vi "Get RemIO Read Scaling Factor.vi"(8 "error in (no error)":errorcluster, 10 "11120 in":refnum<class "11120.lvclass">, 11 "Node Ptr In":T1 format="%.0x") -> (0 "error out":errorcluster, 1 "Scaling Factors":dbl[](array[numeric]), 2 "11120 out":refnum<class "11120.lvclass">, 3 "Node Ptr Out":T1 format="%.0x", 5 "Per Channel?":bool)   [LabVIEW 2019, in "Modules.lvlib" / "11120.lvclass"]
doc: "This VI Returns the scaling factors for REM IO Input Modules"
uses:
  11120.lvclass
  <vilib>/NI VeriStand/Custom Device API/Custom Device Item Ref.ctl
  11120.lvclass/11120.ctl
  6892548b-0d22-43a4-8def-8bcf3b7e9b02.vi
  RemIO Module/Get RemIO Library Path.vi
  <vilib>/NI VeriStand/Custom Device API/Custom Device API.lvlib
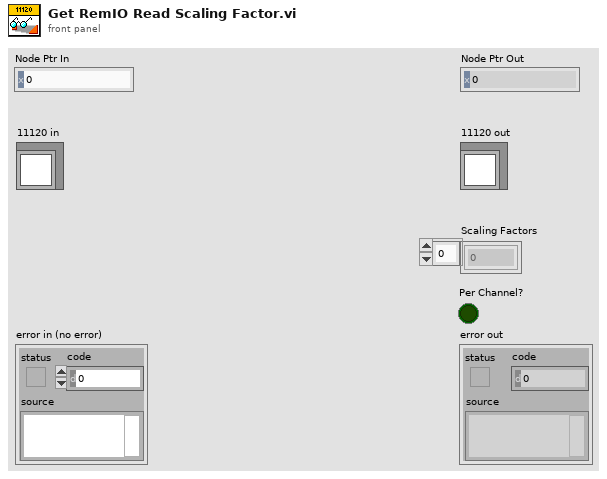
[diagram p1: front panel]
types:
  T1 = typedef "Custom Device API.lvlib/Custom Device Item Ref.ctl" = u64
  T2 = typedef "NI ECAT Remote IO.lvlib/channel number REM-11120.ctl" = u8
  T3 = typedef "NI ECAT Remote IO.lvlib/input filter time REM-11120.ctl" = u8
  T4 = typedef "NI ECAT Remote IO.lvlib/cold junction type REM-11120.ctl" = u8
  T5 = typedef "NI ECAT Remote IO.lvlib/resolution REM-11120.ctl" = u8
  T6 = typedef "NI ECAT Remote IO.lvlib/sensor type REM-11120.ctl" = u8
  T7 = cluster{"channel number":T2, "input filter time":T3, "cold junction type":T4, "resolution":T5, "sensor type":T6}[]
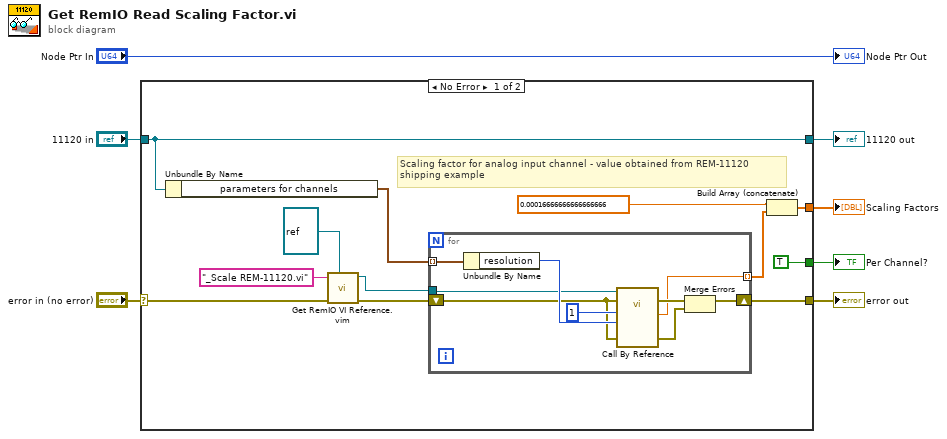
[diagram p0: block diagram]
diagram:
  n1 = case shown="No Error" "error in (no error)" {
    selector: "error in (no error)" -> [w11 w30]
    tunnel: [w18 w30] -> w6
    tunnel: [w17 w29] -> w4
    tunnel: "11120 in" -> [w17 w29]
    tunnel: [w13 _] -> w3
    tunnel: [TRUE _] -> w2
    frame No Error {
      # "Scaling factor for analog input channel - value obtained from REM-11120\nshipping example"
      n2 = Unbundle By Name(w17) -> ("parameters for channels"=w16:T7)
      n3 = call "Get RemIO VI Reference.vim"("name or relative path"="_Scale REM-11120.vi", "error in (no error)"=w11, "type specifier VI Refnum (for type only)"=refnum<vi> refnum) -> ("vi reference"=w8:refnum<vi>, "error out"=w12:errorcluster)  [unwired: 6 in]
      n4 = for {
        shift-right: [w21] -> w18
        shift-left: w12 -> [w22]
        tunnel: [w23] -> w14 mode=indexing
        tunnel: w16 -> [w28] mode=indexing
        tunnel: w8 -> [w20]
        n5 = Unbundle By Name(w28) -> ("resolution"=w25:T5)
        n6 = call-by-ref "?"(reference=w20, error in=w22, 8:"error in (no error)"=w22, "resolution"=w25, "raw data"=u16 1) -> (error out=w26:errorcluster, 0:"error out"=w27:errorcluster, "scaled data"=w23:dbl)  [unwired: 7 in, 1 out]
        n7 = Merge Errors(w26, w27) -> (w21:errorcluster)
      }
      n8 = Build Array (concatenate)(0.00016666666666666666, w14) -> (w13:dbl[])
    }
    frame Error {
    }
  }
  "error out" <- w6
  "11120 out" <- w4
  "Scaling Factors" <- w3
  "Per Channel?" <- w2
  "Node Ptr Out" <- "Node Ptr In"
